vi "Update Matrix.vi"(1 "Older":dbl[][](array[numeric]) format="%.3f", 2 "Current":dbl[](array[numeric]) format="%.3f") -> (0 "New":dbl[][](array[numeric]) format="%.3f")   [LabVIEW 2022 SP3]
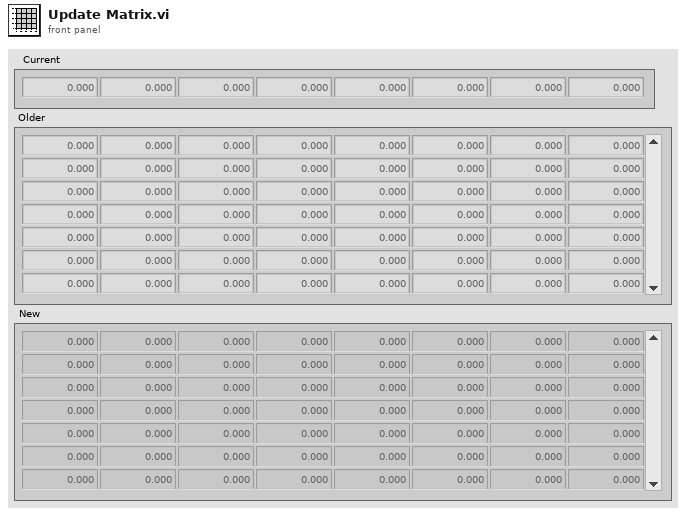
[diagram p1: front panel]
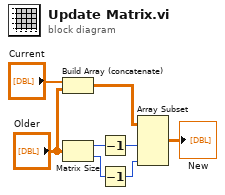
[diagram p0: block diagram]
diagram:
  n1 = Build Array (concatenate)("Current", "Older") -> (w6:dbl[][])
  n2 = Matrix Size(0:"Older") -> (1:w4:i32, 2:w3:i32)
  n3 = Decrement(x=w4) -> (x-1=w1:i32)
  n4 = Decrement(x=w3) -> (x-1=w2:i32)
  n5 = Array Subset(array=w6, length (row)=w1, length (col)=w2) -> (→"New":dbl[][])  [unwired: 2 in]
